vi "runSingleScriptV3.vi"(8 "error in (no error)":errorcluster, 9 "HWLoop":bool, 10 "index":i32, 11 "ExperimentRunner in":refnum<class "ExperimentRunner.lvclass">) -> (0 "error out":errorcluster, 3 "ExperimentRunner out":refnum<class "ExperimentRunner.lvclass">)   [LabVIEW 2011, in "Views.lvlib" / "ExperimentControl.lvlib" / "ExperimentRunner.lvclass"]
uses:
  ExperimentRunner.lvclass
  ExperimentRunner.lvclass/ExperimentRunner.ctl
  Events/ExperimentControlEvents.lvclass
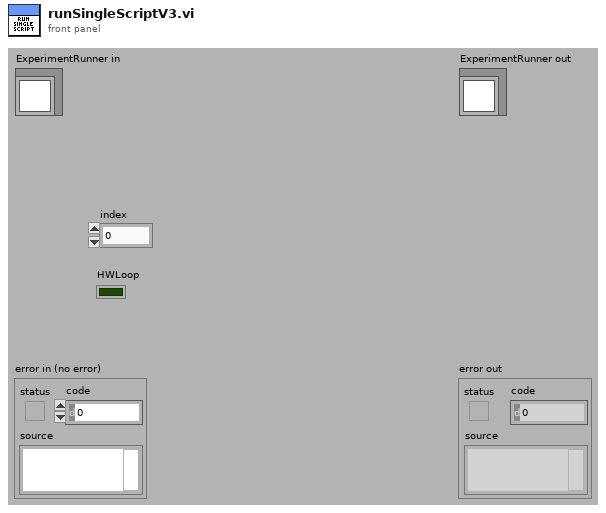
[diagram p1: front panel]
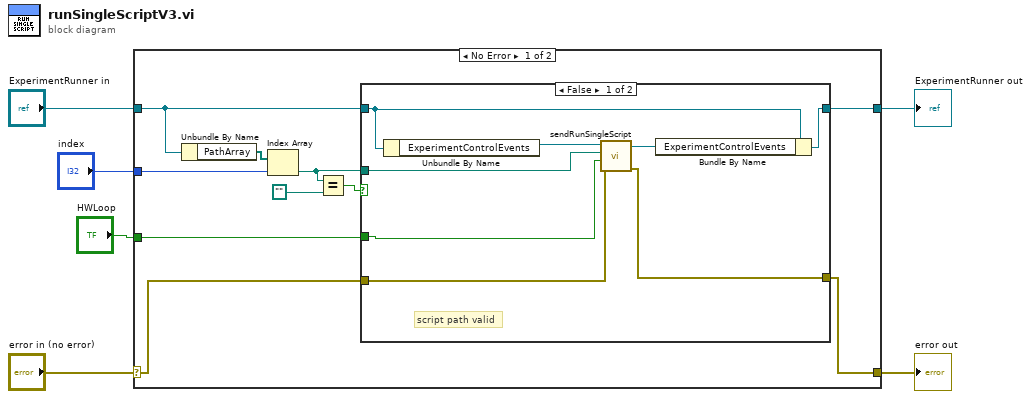
[diagram p0: block diagram]
diagram:
  n1 = case shown="No Error" "error in (no error)" {
    selector: "error in (no error)" -> [w8 w28]
    tunnel: [w7 w28] -> w5
    tunnel: [w11 w27] -> w3
    tunnel: "ExperimentRunner in" -> [w12 w27]
    tunnel: "HWLoop" -> [w10 _]
    tunnel: "index" -> [w15 _]
    frame No Error {
      n2 = Unbundle By Name(w12) -> ("PathArray"=w16:path[])
      n3 = Index Array(array=w16, index=w15) -> (element=w9:path)
      n4 = Equal?(x=w9, y=path "") -> (x = y?=w13:bool)
      n5 = case shown="False" w13 {
        tunnel: w12 -> [w18 w26]
        tunnel: [w17 w26] -> w11
        tunnel: w10 -> [w22 _]
        tunnel: w9 -> [w23 _]
        tunnel: w8 -> [w21 w25]
        tunnel: [w20 w25] -> w7
        frame False {
          # "script path valid"
          n6 = Unbundle By Name(w18) -> ("ExperimentControlEvents"=w24:refnum<class "ExperimentControlEvents.lvclass">)
          n7 = call "sendRunSingleScript.vi"("error in (no error)"=w21, "HWLoop"=w22, "Path"=w23, "ExperimentControlEvents in"=w24) -> ("error out"=w20:errorcluster, "ExperimentControlEvents out"=w19:refnum<class "ExperimentControlEvents.lvclass">)  [unwired: 6 in]
          n8 = Bundle By Name(cluster=w18, "ExperimentControlEvents"=w19) -> (w17:refnum<class "ExperimentRunner.lvclass">)
        }
        frame True {
          # "empty script path"
        }
      }
    }
    frame Error {
    }
  }
  "error out" <- w5
  "ExperimentRunner out" <- w3
